vi "GetFlashFlowRateSetpoint.vi"(7 "Timeout (ms)":u32=2000, 8 "Error In":errorcluster, 11 "Sierra M100 In":refnum<visa-resource-name>) -> (0 "Error Out":errorcluster, 2 "Setpoint (mL/min)":dbl format="%.1f", 3 "Sierra M100 Out":refnum<visa-resource-name>)   [LabVIEW 2012, in "Sierra-M100.lvlib"]
doc: "This VI gets the flow rate setpoint from flash memory in the mass flow controller (MFC). The flash memory is non-volatile. This setpoint is retained during power cycling."
uses:
  Sierra-M100.lvlib
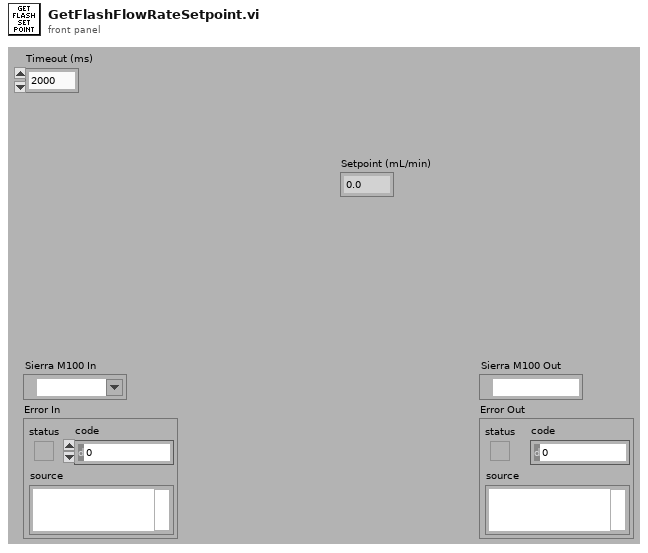
[diagram p1: front panel]
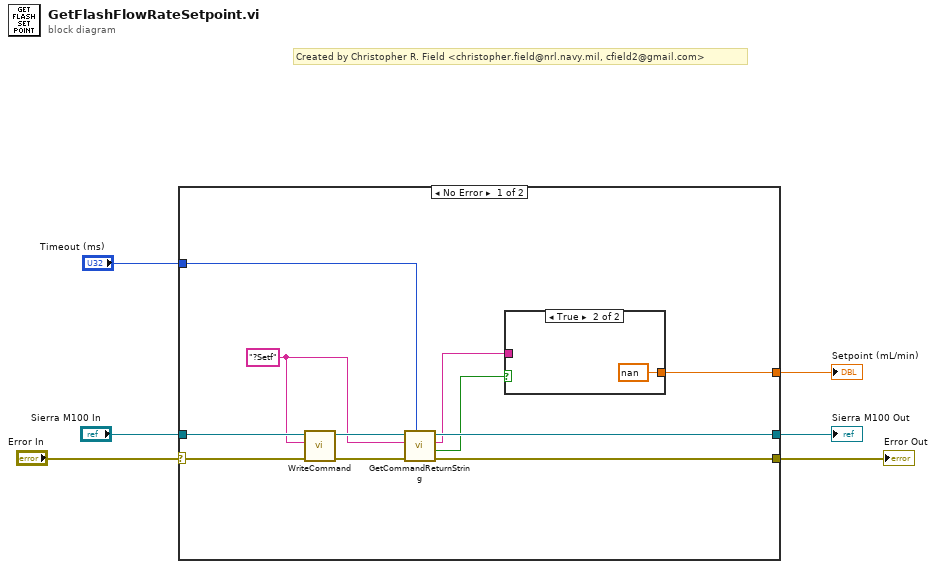
[diagram p0: block diagram]
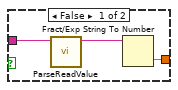
[diagram p2: hidden frame]
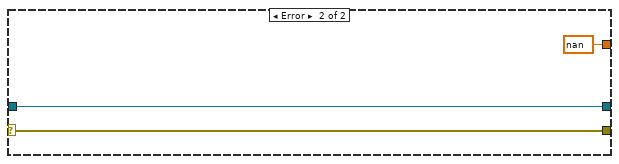
[diagram p3: hidden frame]
diagram:
  # "Created by Christopher R. Field <christopher.field@nrl.navy.mil, cfield2@gmail.com>"
  n1 = case shown="No Error" "Error In" {
    selector: "Error In" -> [w7 w23]
    tunnel: [w17 nan] -> w6
    tunnel: "Sierra M100 In" -> [w16 w24]
    tunnel: "Timeout (ms)" -> [w12 _]
    tunnel: [w11 w24] -> w3
    tunnel: [w10 w23] -> w2
    frame No Error {
      w14 = "?Setf"
      n2 = call "WriteCommand.vi"("Error In"=w7, "Command"=w14, "Sierra M100 In"=w16) -> ("Error Out"=w13:errorcluster, "Sierra M100 Out"=w15:refnum<visa-resource-name>)  [unwired: 5 in, 2 out]
      n3 = call "GetCommandReturnString.vi"("Timeout (ms)"=w12, "Error In"=w13, "Command"=w14, "Sierra M100 In"=w15) -> ("Error Out"=w10:errorcluster, "Timeout?"=w9:bool, "Return String"=w8:string, "Sierra M100 Out"=w11:refnum<visa-resource-name>)  [unwired: 4 in]
      n4 = case shown="True" w9 {
        tunnel: [w20 nan] -> w17
        tunnel: w8 -> [w19 _]
        frame False {
          n5 = call "ParseReadValue.vi"("Read Buffer"=w19) -> ("Value"=w18:string)  [unwired: 10 in]
          n6 = Fract/Exp String To Number(string=w18) -> (number=w20:dbl)  [unwired: 3 in, 1 out]
        }
        frame True {
        }
      }
    }
    frame Error {
    }
  }
  "Sierra M100 Out" <- w3
  "Error Out" <- w2
  "Setpoint (mL/min)" <- w6
